vi "Sensitivity.vi"(0 "TSM context":T1, 5 "Capture Duration (s)":dbl=1.0, 7 "Frequency":dbl=1000.0 format="%#_13g", 9 "dB SPL":dbl=94.0 format="%#_13g") -> (4 "dbSPL":dbl[](array[numeric]), 6 "dB V":dbl[](array[numeric]), 15 "error out":errorcluster)   [LabVIEW 2020]
doc: "Sensitivity Test VI helps to source a known wavefrom (1k Hz) in speaker and capture back the waveform in the DUT and calculate the sensitivity in dBV"
uses:
  <vilib>/NI_TestStand_SemiconductorModule/NI_TestStand_Semiconductor_Module.lvlibp/PinMap/General/SemiconductorModuleContext.ctl
  <vilib>/NI_TestStand_SemiconductorModule/NI_TestStand_Semiconductor_Module.lvlibp/PinMap/TagProvider/TSM_Pin.ctl
  580befc9-3443-43a1-ac84-b2f599be9b8b.vi
  2a88b7c8-4b33-46f4-9564-f1ca216a3d22.vi
  3eea6c6d-84ba-4972-8d7e-d2e842b42d7e.vi
  2c6cc387-348b-4bf2-88b8-472fb92eec90.vi
  76239c40-3b04-4b52-a7f5-0ceeea72be64.vi
  580befc9-3443-43a1-ac84-b2f599be9b8b.vi/e325d36d-f8d5-444c-95fc-e56b98c083a2.vi
  <vilib>/measure/matone.llb/Extract Single Tone Information N Chan.vi
  <vilib>/NI_TestStand_SemiconductorModule/NI_TestStand_Semiconductor_Module.lvlibp/PinMap/General/Publish/PublishDataDoubleFunctionalTest.vi
  <vilib>/NI_TestStand_SemiconductorModule/NI_TestStand_Semiconductor_Module.lvlibp
  <vilib>/measure/NI_MAPro.lvlib
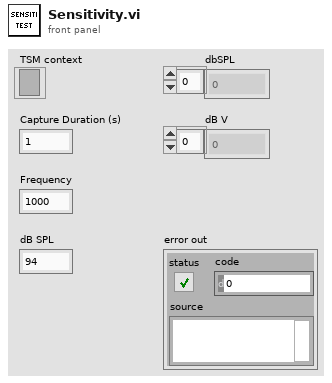
[diagram p1: front panel]
types:
  T1 = typedef "NI_TestStand_Semiconductor_Module.lvlibp/SemiconductorModuleContext.ctl" = refnum<k7>
  T2 = typedef "NI_TestStand_Semiconductor_Module.lvlibp/TSM_Pin.ctl" = tag
  T3 = cluster{"approx freq. (optional)":dbl, "search (+/- % of Fsampl.)":dbl}
  T4 = typedef "TSM DAQmx Multi-Task.ctl" = cluster{"Pin Query Context":refnum<class "MultiplePinMultipleSessionQueryContext.lvclass">, "SSC":T5[], "Site Numbers":i32[], "Pins":tag[]}
  T5 = typedef "SSC DAQmx.ctl" = cluster{"DAQmx Task ":refnum<k21>, "Channels":string, "Channel Lists":string}
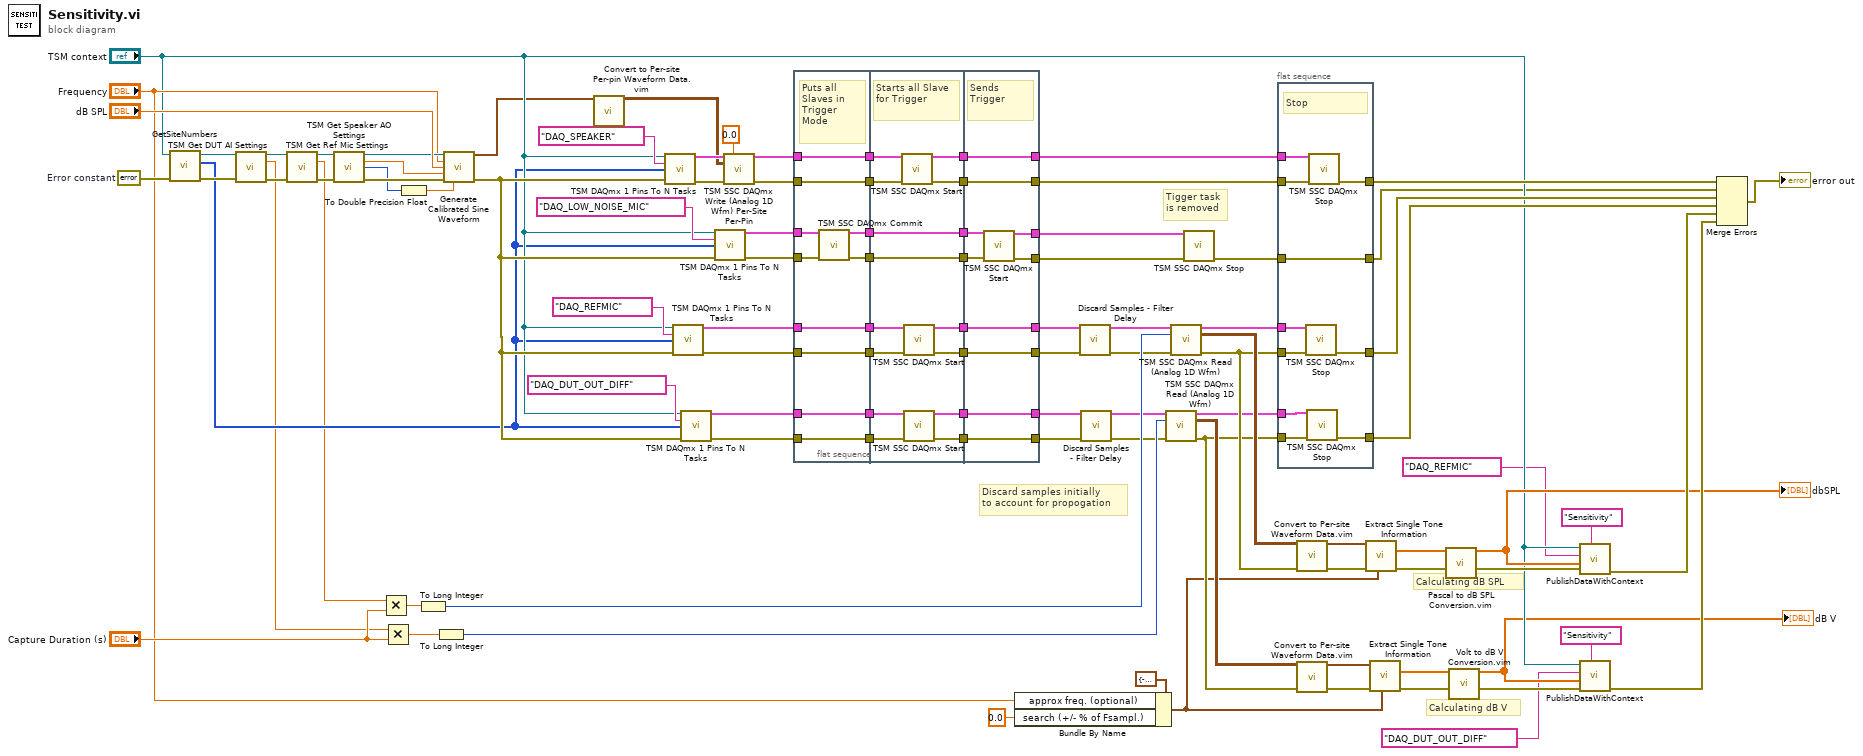
[diagram p0: block diagram]
diagram:
  w98 = errorcluster {"status"=FALSE, "code"=0, "source"=""}  # Error constant
  # "Discard samples initially\nto account for propogation"
  # "Tigger task \nis removed"
  # "Calculating dB SPL"
  # "Calculating dB V"
  n1 = call <vilib>:"GetSiteNumbers.vi"("error in (no error)"=w98, "Semiconductor Module Context"="TSM context") -> ("error out"=w60:errorcluster, "Site Numbers"=w18:i32[], "Semiconductor Module Context Out"=w59:T1)  [unwired: 6 in, 1 out]
  n2 = call "TSM Get DUT AI Settings.vi"("TSM context"=w59, "error in (no error)"=w60) -> ("TSM context Out"=w56:T1, "Sampling Rate (Hz)"=w3:dbl, "error out"=w58:errorcluster)  [unwired: 9 in, 2 out]
  n3 = call "TSM Get Ref Mic Settings.vi"("TSM context"=w56, "error in (no error)"=w58) -> ("TSM context Out"=w55:T1, "Sampling Rate (Hz)"=w4:dbl, "error out"=w57:errorcluster)  [unwired: 8 in, 3 out]
  n4 = call "TSM Get Speaker AO Settings.vi"("TSM context"=w55, "error in (no error)"=w57) -> ("TSM context Out"=w63:T1, "Sampling Rate (Hz)"=w62:dbl, "Samples per channel"=w61:i32, "error out"=w64:errorcluster)  [unwired: 9 in, 1 out]
  n5 = Multiply(x=w4, y="Capture Duration (s)") -> (x*y=w53:dbl)
  n6 = Multiply(x=w3, y="Capture Duration (s)") -> (x*y=w52:dbl)
  n7 = To Double Precision Float(number=w61) -> (double precision float=w65:dbl)
  n8 = To Long Integer(number=w53) -> (32bit integer=w50:i32)
  n9 = To Long Integer(number=w52) -> (32bit integer=w51:i32)
  n10 = call "Generate Calibrated Sine Waveform.vi"("TSM context"=w63, "Frequency (Hz)"="Frequency", "dB SPL"="dB SPL", "Sampling Rate (Hz)"=w62, "error in (no error)"=w64, "Samples per channel"=w65) -> ("Per-Site Waveforms Out"=w14:waveform(dbl)[], "error out"=w29:errorcluster)  [unwired: 7 in, 1 out]
  n11 = call "Convert to Per-site Per-pin Waveform Data.vim"("Waveform In"=w14) -> ("Per Site Per Pin Waveform Out"=w13:waveform(dbl)[][])  [unwired: 14 in]
  n12 = call "TSM DAQmx 1 Pins To N Tasks.vi"("TSM context"="TSM context", "Pins"=tag "DAQ_SPEAKER", "Site Numbers"=w18, "error in"=w29) -> ("DAQ TSM Out"=w92:T4, "error out"=w93:errorcluster)  [unwired: 10 in]
  n13 = call "TSM DAQmx 1 Pins To N Tasks.vi"("TSM context"="TSM context", "Pins"=tag "DAQ_REFMIC", "Site Numbers"=w18, "error in"=w29) -> ("DAQ TSM Out"=w85:T4, "error out"=w89:errorcluster)  [unwired: 10 in]
  n14 = call "TSM DAQmx 1 Pins To N Tasks.vi"("TSM context"="TSM context", "Pins"=tag "DAQ_DUT_OUT_DIFF", "Site Numbers"=w18, "error in"=w29) -> ("DAQ TSM Out"=w84:T4, "error out"=w88:errorcluster)  [unwired: 10 in]
  n15 = call "TSM DAQmx 1 Pins To N Tasks.vi"("TSM context"="TSM context", "Pins"=tag "DAQ_LOW_NOISE_MIC", "Site Numbers"=w18, "error in"=w29) -> ("DAQ TSM Out"=w23:T4, "error out"=w28:errorcluster)  [unwired: 10 in]
  n16 = call "TSM SSC DAQmx Write (Analog 1D Wfm) Per-Site Per-Pin.vi"("DAQ TSM in"=w92, "Idle Channel Value (0)"=0.0, "Per-Site Per-Pin Waveforms in"=w13, "error in"=w93) -> ("DAQ TSM Out"=w90:T4, "error out"=w91:errorcluster)  [unwired: 10 in]
  n17 = flat-sequence {
    tunnel: w84 -> [w103]
    tunnel: w85 -> [w104]
    tunnel: w90 -> [w105]
    tunnel: w91 -> [w106]
    tunnel: w88 -> [w107]
    tunnel: w89 -> [w108]
    tunnel: [w108] -> w42
    tunnel: [w107] -> w41
    tunnel: [w106] -> w40
    tunnel: [w105] -> w39
    tunnel: [w104] -> w38
    tunnel: [w103] -> w37
    tunnel: w28 -> [w102]
    tunnel: [w101] -> w27
    tunnel: w23 -> [w100]
    tunnel: [w99] -> w21
    tunnel: w42 -> [w122]
    tunnel: w41 -> [w121]
    tunnel: w40 -> [w112]
    tunnel: w39 -> [w110]
    tunnel: w38 -> [w118]
    tunnel: w37 -> [w117]
    tunnel: [w111] -> w36
    tunnel: [w109] -> w35
    tunnel: [w120] -> w34
    tunnel: [w119] -> w33
    tunnel: [w116] -> w32
    tunnel: [w115] -> w31
    tunnel: w27 -> [w114]
    tunnel: [w114] -> w26
    tunnel: [w113] -> w22
    tunnel: w21 -> [w113]
    tunnel: [w127] -> w10
    tunnel: [w128] -> w6
    tunnel: [w129] -> w12
    tunnel: [w130] -> w8
    tunnel: [w131] -> w86
    tunnel: [w132] -> w87
    tunnel: w36 -> [w132]
    tunnel: w35 -> [w131]
    tunnel: w34 -> [w130]
    tunnel: w33 -> [w129]
    tunnel: w32 -> [w128]
    tunnel: w31 -> [w127]
    tunnel: w26 -> [w126]
    tunnel: [w125] -> w25
    tunnel: w22 -> [w124]
    tunnel: [w123] -> w20
    frame #0 {
      # "Puts all Slaves in Trigger Mode"
      n18 = call "TSM SSC DAQmx Commit.vi"("TSM DAQmx In"=w100, "error in (no error)"=w102) -> ("TSM DAQmx Out"=w99:T4, "error out"=w101:errorcluster)  [unwired: 12 in]
    }
    frame #1 {
      # "Starts all Slave for Trigger"
      n19 = call "TSM SSC DAQmx Start.vi"("TSM DAQmx In"=w110, "error in (no error)"=w112) -> ("TSM DAQmx Out"=w109:T4, "error out"=w111:errorcluster)  [unwired: 12 in]
      n20 = call "TSM SSC DAQmx Start.vi"("TSM DAQmx In"=w118, "error in (no error)"=w122) -> ("TSM DAQmx Out"=w116:T4, "error out"=w120:errorcluster)  [unwired: 12 in]
      n21 = call "TSM SSC DAQmx Start.vi"("TSM DAQmx In"=w117, "error in (no error)"=w121) -> ("TSM DAQmx Out"=w115:T4, "error out"=w119:errorcluster)  [unwired: 12 in]
    }
    frame #2 {
      # "Sends Trigger"
      n22 = call "TSM SSC DAQmx Start.vi"("TSM DAQmx In"=w124, "error in (no error)"=w126) -> ("TSM DAQmx Out"=w123:T4, "error out"=w125:errorcluster)  [unwired: 12 in]
    }
  }
  n23 = Bundle By Name(cluster=T3 {"approx freq. (optional)"=-1.0, "search (+/- % of Fsampl.)"=5.0} ("advanced search"), "approx freq. (optional)"="Frequency", "search (+/- % of Fsampl.)"=0.0) -> (w46:T3)
  n24 = call "Discard Samples - Filter Delay.vi"("DAQ TSM in"=w6, "error in"=w8) -> ("DAQ TSM Out"=w5:T4, "error out"=w7:errorcluster)  [unwired: 12 in]
  n25 = call "Discard Samples - Filter Delay.vi"("DAQ TSM in"=w10, "error in"=w12) -> ("DAQ TSM Out"=w9:T4, "error out"=w11:errorcluster)  [unwired: 12 in]
  n26 = call "TSM SSC DAQmx Read (Analog 1D Wfm).vi"("DAQ TSM in"=w9, "Samples to read"=w51, "error in"=w11) -> ("DAQ TSM Out"=w78:T4, "Per-Site Per-Pin Waveforms Out"=w82:waveform(dbl)[][], "error out"=w77:errorcluster)  [unwired: 10 in]
  n27 = call "TSM SSC DAQmx Read (Analog 1D Wfm).vi"("DAQ TSM in"=w5, "Samples to read"=w50, "error in"=w7) -> ("DAQ TSM Out"=w81:T4, "Per-Site Per-Pin Waveforms Out"=w83:waveform(dbl)[][], "error out"=w79:errorcluster)  [unwired: 10 in]
  n28 = call "TSM SSC DAQmx Stop.vi"("TSM DAQmx In"=w20, "error in (no error)"=w25) -> ("error out"=w24:errorcluster)  [unwired: 12 in, 1 out]
  n29 = flat-sequence {
    tunnel: w87 -> [w142]
    tunnel: [w141] -> w72
    tunnel: w86 -> [w140]
    tunnel: w79 -> [w139]
    tunnel: [w138] -> w71
    tunnel: w77 -> [w137]
    tunnel: [w136] -> w70
    tunnel: w78 -> [w135]
    tunnel: w81 -> [w134]
    tunnel: w24 -> [w133]
    tunnel: [w133] -> w17
    frame #0 {
      # "Stop"
      n30 = call "TSM SSC DAQmx Stop.vi"("TSM DAQmx In"=w134, "error in (no error)"=w139) -> ("error out"=w138:errorcluster)  [unwired: 12 in, 1 out]
      n31 = call "TSM SSC DAQmx Stop.vi"("TSM DAQmx In"=w135, "error in (no error)"=w137) -> ("error out"=w136:errorcluster)  [unwired: 12 in, 1 out]
      n32 = call "TSM SSC DAQmx Stop.vi"("TSM DAQmx In"=w140, "error in (no error)"=w142) -> ("error out"=w141:errorcluster)  [unwired: 12 in, 1 out]
    }
  }
  n33 = call "Convert to Per-site Waveform Data.vim"("Per-Site Per-Pin Waveform In"=w83) -> ("Per-Site Waveform Out"=w80:waveform(dbl)[])  [unwired: 14 in]
  n34 = call "Convert to Per-site Waveform Data.vim"("Per-Site Per-Pin Waveform In"=w82) -> ("Per-Site Waveform Out"=w43:waveform(dbl)[])  [unwired: 14 in]
  n35 = call-poly <vilib>:"Extract Single Tone Information.vi"("advanced search"=w46, "error in (no error)"=w79, "time signals in"=w80) -> ("error out"=w75:errorcluster, "detected amplitudes"=w45:dbl[])  [unwired: 3 in, 4 out]
  n36 = call-poly <vilib>:"Extract Single Tone Information.vi"("advanced search"=w46, "error in (no error)"=w77, "time signals in"=w43) -> ("error out"=w76:errorcluster, "detected amplitudes"=w16:dbl[])  [unwired: 3 in, 4 out]
  n37 = call "Pascal to dB SPL Conversion.vim"("Pascals"=w45) -> ("dbSPL"=w44:dbl[])  [unwired: 14 in]
  "dbSPL" <- w44
  n38 = call "Volt to dB V Conversion.vim"("Voltage"=w16) -> ("dB V"=w15:dbl[])  [unwired: 14 in]
  "dB V" <- w15
  n39 = call-poly <vilib>:"PublishDataWithContext.vi"("Published Data Id"="Sensitivity", "error in (no error)"=w75, "Data In"=w44, "Pin"=T2 "DAQ_REFMIC", "Semiconductor Module Context"="TSM context") -> ("error out"=w69:errorcluster)  [unwired: 5 in, 1 out]
  n40 = call-poly <vilib>:"PublishDataWithContext.vi"("Published Data Id"="Sensitivity", "error in (no error)"=w76, "Data In"=w15, "Pin"=T2 "DAQ_DUT_OUT_DIFF", "Semiconductor Module Context"="TSM context") -> ("error out"=w68:errorcluster)  [unwired: 5 in, 1 out]
  n41 = Merge Errors(w72, w17, w71, w70, w69, w68) -> (→"error out":errorcluster)
